vi "calib.vi"() -> ()   [LabVIEW 2015]
uses:
  phlib.dll
panel:
  out "Returncode":i32
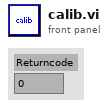
[diagram p1: front panel]
types:
  T1 = cluster{"initialized":bool, "devidx":i32, "Ch0 Level":i32, "Ch0 ZeroX":i32, "Ch1 Level":i32, "Ch1 ZeroX":i32, "sync rate":i32, "resolution":i32, "acq time":i32, "acq rate":i32, "# bins":u32, "Bin size":enum16{"1", "2", "4", "8", "16", "32", "64", "128"}, "min photons":u32, "truncate":u32}
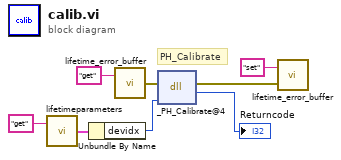
[diagram p0: block diagram]
diagram:
  # "PH_Calibrate"
  n1 = call "lifetimeparameters.vi"("command"="get") -> ("Params out"=w6:T1)  [unwired: 1 in]
  n2 = Unbundle By Name(w6) -> ("devidx"=w5:i32)
  n3 = call "lifetime_error_buffer.vi"("command"="get") -> ("error out"=w2:errorcluster)  [unwired: 1 in]
  n4 = dll-call lib="phlib.dll" fn="_PH_Calibrate@4"(error in=w2, "devidx"=w5) -> (error out=w1:errorcluster, →"Returncode":i32)  [unwired: 3 in, 1 out]
  n5 = call "lifetime_error_buffer.vi"("error in"=w1, "command"="set") -> ()  [unwired: 1 out]
